vi "MFCquery.vi"(8 "error in (no error)":errorcluster, 9 "cmd":string, 10 "Device ID's":string[](array[string]), 11 "VISA Refnum in":refnum<visa-resource-name>) -> (0 "error out":errorcluster, 2 "Array":string[](array[string]), 3 "VISA Refnum out":refnum<visa-resource-name>)   [LabVIEW 2020, in "MFC.lvclass"]
uses:
  MFC/MFC.lvclass
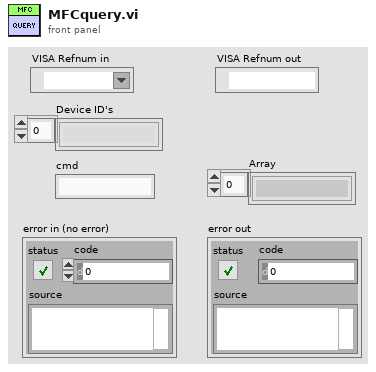
[diagram p1: front panel]
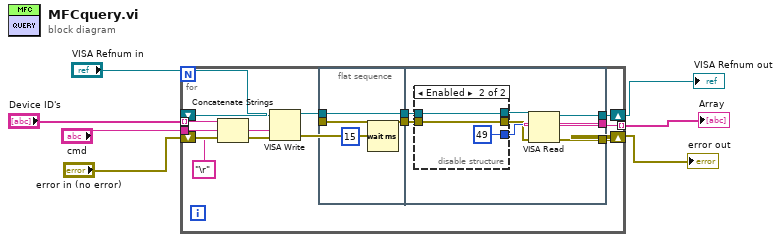
[diagram p0: block diagram]
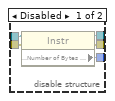
[diagram p2: hidden frame]
diagram:
  n1 = for {
    tunnel: "Device ID's" -> [w11] mode=indexing
    shift-right: [w17] -> w5
    shift-left: "error in (no error)" -> [w18]
    shift-right: [w15] -> w6
    shift-left: "VISA Refnum in" -> [w16]
    tunnel: [w14] -> w7 mode=indexing
    tunnel: "cmd" -> [w9]
    n2 = Concatenate Strings(w11, w9, "\r" ("string")) -> (w10:string)
    n3 = VISA Write(VISA resource name=w16, write buffer=w10, error in (no error)=w18) -> (VISA resource name out=w20:refnum<visa-resource-name>, error out=w19:errorcluster)  [unwired: 1 out]
    n4 = flat-sequence {
      tunnel: w19 -> [w22]
      tunnel: w20 -> [w23]
      tunnel: [w23] -> w13
      tunnel: [w22] -> w12
      tunnel: [w26] -> w17
      tunnel: [w25] -> w15
      tunnel: [w24] -> w14
      tunnel: w13 -> [w31]
      tunnel: w12 -> [w27]
      frame #0 {
        n5 = Wait (ms)(milliseconds to wait=u32 15) -> ()  [unwired: 1 out]
      }
      frame #1 {
        n6 = disable-structure shown="Enabled" {
          disable-tunnel: w31 -> [w36 w39]
          disable-tunnel: [w35 w39] -> w30
          disable-tunnel: [w34 u32 49 ("Bytes at Port")] -> w29
          disable-tunnel: [w33 w38] -> w28
          disable-tunnel: w27 -> [w32 w38]
          frame Disabled {
            n7 = property class="Instr"(reference=w36, error in=w32) -> (reference out=w35:refnum<visa-resource-name>, error out=w33:errorcluster, "Serial Settings:Number of Bytes at Serial Port"=w34:u32)
          }
          frame Enabled {
          }
        }
        n8 = VISA Read(VISA resource name=w30, byte count=w29, error in (no error)=w28) -> (VISA resource name out=w25:refnum<visa-resource-name>, read buffer=w24:string, error out=w26:errorcluster)  [unwired: 1 out]
      }
    }
  }
  "Array" <- w7
  "VISA Refnum out" <- w6
  "error out" <- w5
